vi "GenRainbow.vi"(6 "Reset":bool, 11 "NumLeds":i32) -> (3 "Rainbow":u32[](array[colorbox]))   [LabVIEW 2025, in "ArduinoSerialBling.lvlib"]
uses:
  ArduinoSerialBling.lvlib
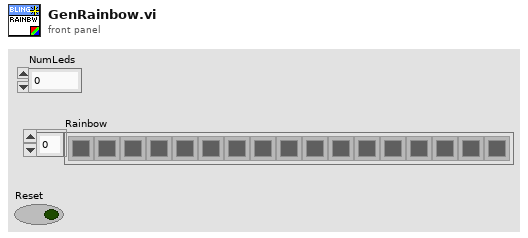
[diagram p1: front panel]
types:
  T1 = enum32{"Gray", "Binary", "Gradient", "Rainbow", "Temperature"}
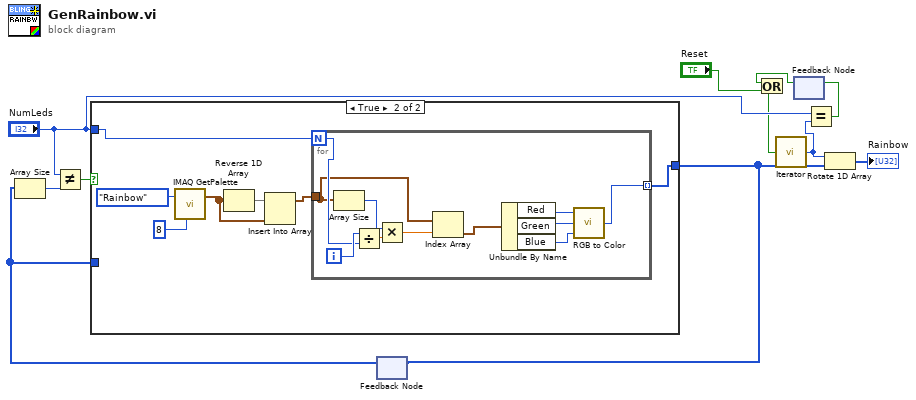
[diagram p0: block diagram]
diagram:
  n1 = feedback #1() -> (w9:u32[])  [unwired: 1 in]
  n2 = Array Size(array=w9) -> (size(s)=w11:i32)
  n3 = Not Equal?(x="NumLeds", y=w11) -> (x != y?=w10:bool)
  n4 = case shown="True" w10 {
    tunnel: "NumLeds" -> [_ w13]
    tunnel: [w12 w14] -> w7
    tunnel: w9 -> [w12 _]
    frame False {
    }
    frame True {
      n5 = call "IMAQ GetPalette"("Palette Number (gray)"=T1."Rainbow", "Bit Depth"=u32 8) -> ("Color Palette"=w16:cluster{"Red":u8, "Green":u8, "Blue":u8}[])  [unwired: 3 in, 1 out]
      n6 = Reverse 1D Array(array=w16) -> (reversed array=w17:cluster{"Red":u8, "Green":u8, "Blue":u8}[])
      n7 = Insert Into Array(array=w17, new element=w16) -> (w15:cluster{"Red":u8, "Green":u8, "Blue":u8}[])  [unwired: 1 in]
      n8 = for {
        N: w13 -> [w29]
        tunnel: [w20] -> w14 mode=indexing
        tunnel: w15 -> [w25]
        i -> [w30]
        n9 = Array Size(array=w25) -> (size(s)=w27:i32)
        n10 = Divide(x=w30, y=w29) -> (x/y=w28:dbl)
        n11 = Multiply(x=w27, y=w28) -> (x*y=w26:dbl)
        n12 = Index Array(array=w25, index=w26) -> (element=w24:cluster{"Red":u8, "Green":u8, "Blue":u8})
        n13 = Unbundle By Name(w24) -> ("Red"=w23:u8, "Green"=w22:u8, "Blue"=w21:u8)
        n14 = call <vilib>:"RGB to Color.vi"("B"=w21, "G"=w22, "R"=w23) -> ("Color"=w20:u32)
      }
    }
  }
  n15 = feedback-in #1(w7) -> ()
  n16 = feedback #2() -> (w3:bool)  [unwired: 1 in]
  n17 = Or(x=w3, y="Reset") -> (x .or. y?=w2:bool)
  n18 = call "Iterator.vi"("Reset"=w2) -> ("i"=w6:i32)
  n19 = Equal?(x="NumLeds", y=w6) -> (x = y?=w4:bool)
  n20 = feedback-in #2(w4) -> ()
  n21 = Rotate 1D Array(1:w7, 2:w6) -> (0:→"Rainbow":u32[])
